vi "ReadChannelStatusFPGA.vi"(7 "IEPE settling blocks":i32=20, 8 "error in":errorcluster, 10 "Wfm Data":waveform(sgl)[](array[waveform]), 11 "Dynamic FPGA VI Reference":T1) -> (0 "error out":errorcluster, 2 "Wfm Data":waveform(sgl)[](array[waveform]), 3 "Dynamic FPGA VI Reference":T1)   [LabVIEW 2017, in "cRIOWfmLib.lvlib"]
doc: "This VI sets the host application's data buffer size, which is critical for maximum data throughput. This buffer is responsible for receiving data coming from the FPGA DMA FIFO. For the continuous case the buffer size should be many times larger than your read size. In the finite case, the timing VIs automatically call this VI and set the buffer size equal to the number of samples in the acquisition."
uses:
  <vilib>/addons/InsightCM/Devices/Shared/Cms/cRIOWfmAcq/cRIOWfmLib.lvlib
  <vilib>/addons/InsightCM/Devices/Shared/Cms/cRIOWfmAcq/subVIs/RIO Wfm Cust Ctrls/rwfm_DynamicFPGAref2.ctl
  <vilib>/addons/InsightCM/Devices/Shared/Cms/cRIOWfmAcq/subVIs/stretchState.ctl
  <vilib>/Utility/error.llb/Error Cluster From Error Code.vi
  <vilib>/rvi/errors/niLvFpgaAdjustHostInterfaceError.vi
  <vilib>/rvi/interface/nirviReadWriteControl/nirviReadWriteControl.xnode
  <vilib>/addons/InsightCM/Utilities/ChannelStatus/ChannelStatus.lvlib
  NiFpgaLv.dll
  <vilib>/rvi/interface/Simulation/niFpgaSimulationCallBeginRW.vi
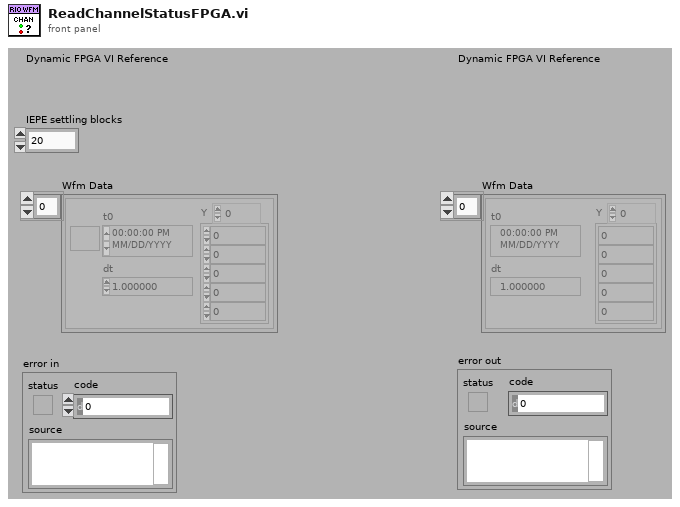
[diagram p1: front panel]
types:
  T1 = typedef "cRIOWfmLib.lvlib/rwfm_DynamicFPGAref2.ctl" = refnum<k20>
  T2 = typedef "cRIOWfmLib.lvlib/stretchState.ctl" = cluster{"input":bool, "output":bool, "pulse count":i32}
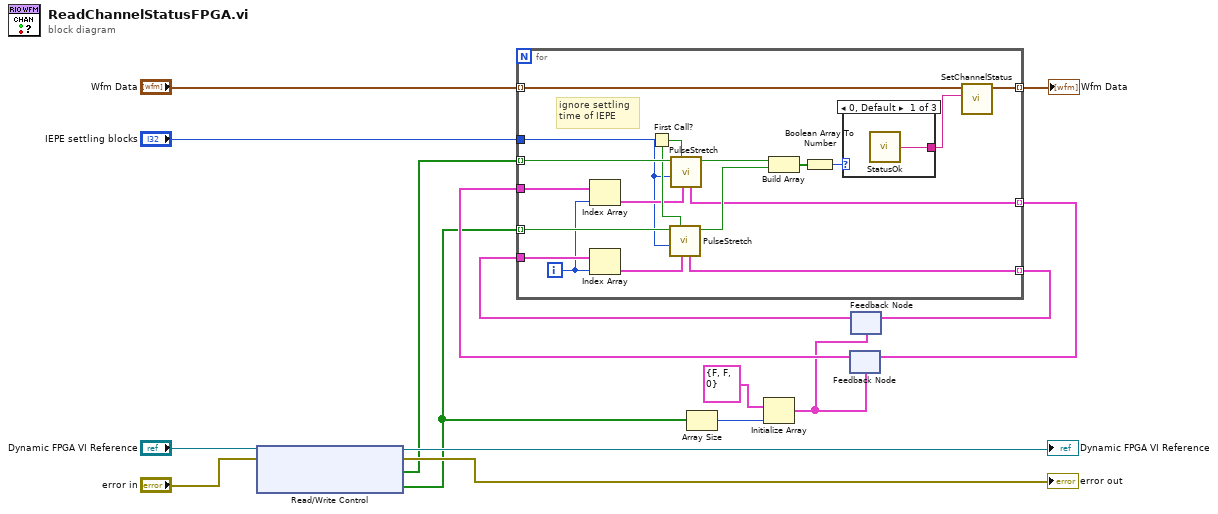
[diagram p0: block diagram]
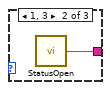
[diagram p2: hidden frame]
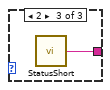
[diagram p3: hidden frame]
diagram:
  n1 = xnode "Read/Write Control"("FPGA VI Reference In"="Dynamic FPGA VI Reference", "error in"="error in") -> ("FPGA VI Reference Out"=→"Dynamic FPGA VI Reference":T1, "error out"=→"error out":errorcluster, "Open Loop Chan Array"=w11:bool[], "Short Circuit Chan Array"=w5:bool[])
  n2 = Array Size(array=w5) -> (size(s)=w4:i32)
  n3 = Initialize Array(T2 {"input"=FALSE, "output"=FALSE, "pulse count"=0} ("element"), w4) -> (w2:T2[])
  n4 = feedback #1(w2) -> (w6:T2[])
  n5 = feedback #2(w2) -> (w8:T2[])
  n6 = for {
    tunnel: "Wfm Data" -> [w18] mode=indexing
    tunnel: w11 -> [w34] mode=indexing
    tunnel: w5 -> [w32] mode=indexing
    tunnel: [w17] -> w10 mode=indexing
    tunnel: [w29] -> w9 mode=indexing
    tunnel: [w28] -> w7 mode=indexing
    tunnel: w8 -> [w27]
    tunnel: w6 -> [w25]
    tunnel: "IEPE settling blocks" -> [w22]
    i -> [w23]
    # "ignore settling \ntime of IEPE"
    n7 = Index Array(array=w25, index=w23) -> (element=w24:T2)
    n8 = Index Array(array=w27, index=w23) -> (element=w26:T2)
    n9 = First Call?() -> (First Call?: T/F=w30:bool)
    n10 = call <vilib>:"PulseStretch.vi"("state in"=w26, "Reset"=w30, "Pulse Width"=w22, "Input"=w32) -> ("Output"=w31:bool, "state out"=w29:T2)  [unwired: 6 in]
    n11 = call <vilib>:"PulseStretch.vi"("state in"=w24, "Reset"=w30, "Pulse Width"=w22, "Input"=w34) -> ("Output"=w33:bool, "state out"=w28:T2)  [unwired: 6 in]
    n12 = Build Array(w33, w31) -> (w21:bool[])
    n13 = Boolean Array To Number(Boolean array=w21) -> (number=w20:u32)
    n14 = case shown="0, Default" w20 {
      tunnel: [w35 w36 w37] -> w19
      frame 0, Default {
        n15 = call <vilib>:"StatusOk.vi"() -> ("status"=w35:string)  [unwired: 5 in]
      }
      frame 1, 3 {
        n16 = call <vilib>:"StatusOpen.vi"() -> ("status"=w36:string)  [unwired: 5 in]
      }
      frame 2 {
        n17 = call <vilib>:"StatusShort.vi"() -> ("status"=w37:string)  [unwired: 5 in]
      }
    }
    n18 = call <vilib>:"SetChannelStatus.vi"("Channel Status"=w19, "Waveform in"=w18) -> ("Waveform out"=w17:waveform(sgl))  [unwired: 8 in, 1 out]
  }
  "Wfm Data" <- w10
  n19 = feedback-in #1(w7) -> ()
  n20 = feedback-in #2(w9) -> ()
